vi "Get Item Ref.vi"(8 "error in (no error)":errorcluster caption="错误输入（无错误）", 11 "ToolStripLabel 输入":refnum<class "ToolStripLabel.lvclass"> caption="DNL_LabVIEW Object in") -> (0 "error out":errorcluster caption="错误输出", 2 "ItemRef":refnum<k24>, 3 "ToolStripLabel 输出":refnum<class "ToolStripLabel.lvclass"> caption="DNL_LabVIEW Object out")   [LabVIEW 2013, in "ToolStripLabel.lvclass"]
uses:
  ToolStripLabel.lvclass
  System.Windows.Forms
  ToolStripLabel.lvclass/ToolStripLabel.ctl
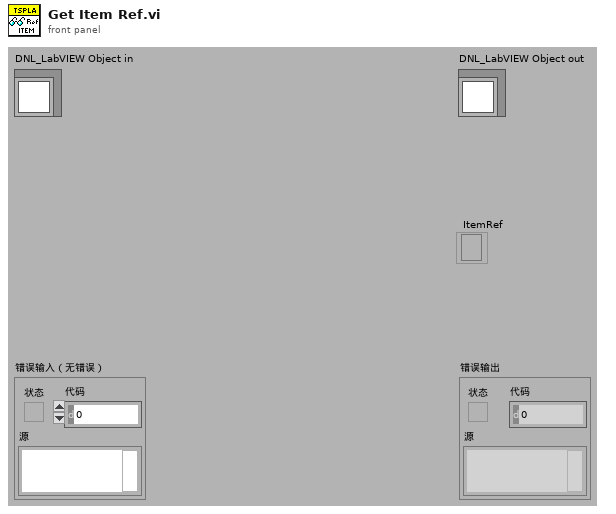
[diagram p1: front panel]
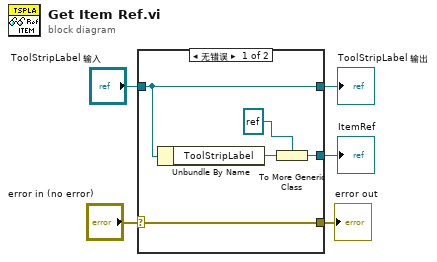
[diagram p0: block diagram]
diagram:
  n1 = case shown="无错误" "error in (no error)" {
    selector: "error in (no error)" -> [w10 w12]
    tunnel: [w10 w12] -> w4
    tunnel: [w9 w11] -> w2
    tunnel: "ToolStripLabel 输入" -> [w9 w11]
    tunnel: [w6 _] -> w1
    frame No Error {
      n2 = Unbundle By Name(w9) -> ("ToolStripLabel"=w8:refnum<k24>)
      n3 = To More Generic Class(target class=refnum<k24> refnum ("value"), reference=w8) -> (generic class reference=w6:refnum<k24>)
    }
    frame Error {
    }
  }
  "error out" <- w4
  "ToolStripLabel 输出" <- w2
  "ItemRef" <- w1
